vi "delete Read Node from VIPB.vi"(8 "error in":errorcluster, 10 "VIPB File Path":path) -> (0 "error out":errorcluster, 2 "Package_LabVIEW_Version":string)   [LabVIEW 2019]
uses:
  <vilib>/xml/Close Reference(Node).vi
  <vilib>/xml/NI_XML.lvlib
  <resource>/objmgr/DOMUserDefRef.rc
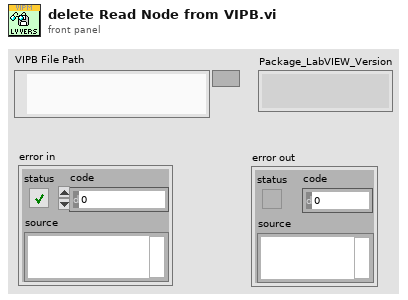
[diagram p1: front panel]
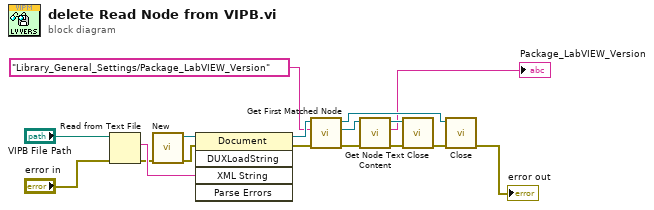
[diagram p0: block diagram]
diagram:
  n1 = Read from Text File(file (use dialog)="VIPB File Path", error in="error in") -> (text=w15:string, error out=w9:errorcluster)  [unwired: 2 in, 2 out]
  n2 = call <vilib>:"New.vi"("error in (no error)"=w9) -> ("error out"=w8:errorcluster, "DOM document out"=w16:refnum<k20>)  [unwired: 7 in]
  n3 = invoke class="Document" method="DUXLoadString"(reference=w16, error in=w8, "XML String"=w15) -> (reference out=w14:refnum<k20>, error out=w7:errorcluster)  [unwired: 2 in, 3 out]
  n4 = call <vilib>:"Get First Matched Node.vi"("error in (no error)"=w7, "XPath expression"="Library_General_Settings/Package_LabVIEW_Version", "node in"=w14) -> ("error out"=w6:errorcluster, "node result"=w12:refnum<k20>, "node out"=w13:refnum<k20>)  [unwired: 6 in]
  n5 = call <vilib>:"Get Node Text Content.vi"("error in (no error)"=w6, "node in"=w12) -> ("error out"=w5:errorcluster, "node text"=→"Package_LabVIEW_Version":string, "node out"=w11:refnum<k20>)  [unwired: 7 in]
  n6 = call-poly <vilib>:"Close.vi"("error in (no error)"=w5, "node"=w11) -> ("error out"=w4:errorcluster)  [unwired: 7 in]
  n7 = call-poly <vilib>:"Close.vi"("error in (no error)"=w4, "node"=w13) -> ("error out"=→"error out":errorcluster)  [unwired: 7 in]
